vi "Fetch PRACH Sequence Index Preamble Results.vi"(8 "error in (no error)":errorcluster, 9 "Preamble (1)":T1=1, 10 "Instance (1)":T2=1, 11 "VISA resource name":refnum<visa-resource-name>) -> (0 "error out":errorcluster, 1 "Result":i32, 2 "Reliability":i32, 3 "VISA resource name out":refnum<visa-resource-name>)   [LabVIEW 2020, in "Rohde&Schwarz CMWXP NR FR1 Measurement.lvlib"]
doc: "Returns the automatically detected or manually configured sequence index for a selected preamble of multi-preamble measurements.\n\nAttribute:\nRSCMWXPNRFR1M_ATTR_FETCH_PRACH_SEQUENCE_INDEX_PREAMBLE_RESULTS\n\nRemote-control command:\nFETCh:NRSub:MEAS<i>:PRACh:MODulation:DSINdex:PREamble<Number>?"
uses:
  <instrlib>/Rohde&Schwarz CMWXP NR FR1 Measurement/Rohde&Schwarz CMWXP NR FR1 Measurement.lvlib
  <instrlib>/Rohde&Schwarz CMWXP NR FR1 Measurement/Private/_Instance.ctl
  <instrlib>/Rohde&Schwarz CMWXP NR FR1 Measurement/Private/_Preamble.ctl
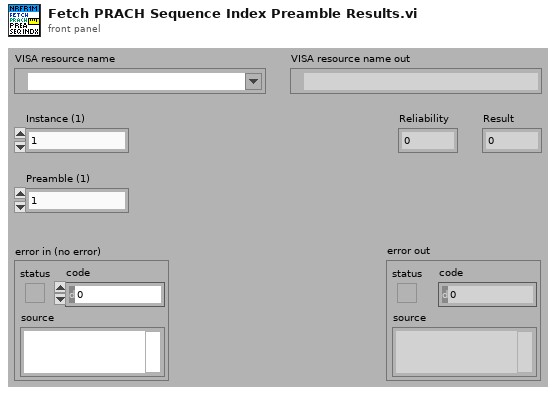
[diagram p1: front panel]
types:
  T1 = typedef "Rohde&Schwarz CMWXP NR FR1 Measurement.lvlib/_Preamble.ctl" = i32
  T2 = typedef "Rohde&Schwarz CMWXP NR FR1 Measurement.lvlib/_Instance.ctl" = i32
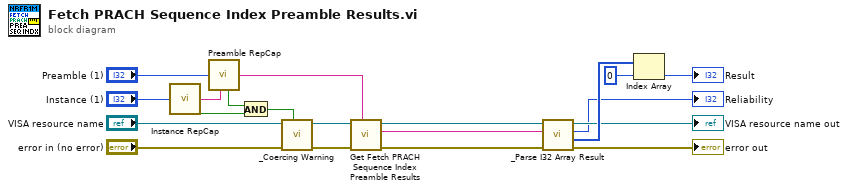
[diagram p0: block diagram]
diagram:
  n1 = call <instrlib>:"Instance RepCap.vi"("Instance In"="Instance (1)") -> ("In Range?"=w19:bool, "RepCap Identifier Out"=w20:string)  [unwired: 1 in]
  n2 = call <instrlib>:"Preamble RepCap.vi"("Preamble In"="Preamble (1)", "RepCap String In (\"\")"=w20) -> ("In Range?"=w18:bool, "RepCap Identifier Out"=w10:string)
  n3 = And(x=w18, y=w19) -> (x .and. y?=w17:bool)
  n4 = call <instrlib>:"_Coercing Warning.vi"("In Range?"=w17, "error in (no error)"="error in (no error)", "VISA resource name"="VISA resource name") -> ("error out"=w11:errorcluster, "VISA resource name out"=w12:refnum<visa-resource-name>)  [unwired: 7 in]
  n5 = call "Get Fetch PRACH Sequence Index Preamble Results"("Repeated Capabilities"=w10, "error in (no error)"=w11, "instrument handle"=w12) -> ("error out"=w5:errorcluster, "Fetch PRACH Sequence Index Preamble Results"=w6:string, "instrument handle out"=w7:refnum<visa-resource-name>)  [unwired: 6 in]
  n6 = call <instrlib>:"_Parse I32 Array Result.vi"("error in (no error)"=w5, "Input String"=w6, "VISA resource name"=w7) -> ("error out"=→"error out":errorcluster, "Results"=w9:i32[], "Reliability"=→"Reliability":i32, "VISA resource name out"=→"VISA resource name out":refnum<visa-resource-name>)  [unwired: 5 in]
  n7 = Index Array(array=w9, index=0) -> (element=→"Result":i32)
